vi "Config - Query.vi"(8 "error in (no error)":errorcluster, 11 "Config Records":T1[](array[typedef])) -> (0 "error out":errorcluster, 3 "Timing Data":u32[](array[numeric]))   [LabVIEW 2017]
doc: "Provide query timing data operation for configuration database process.\n[Covers: SD5]"
uses:
  Controls/Config Record.ctl
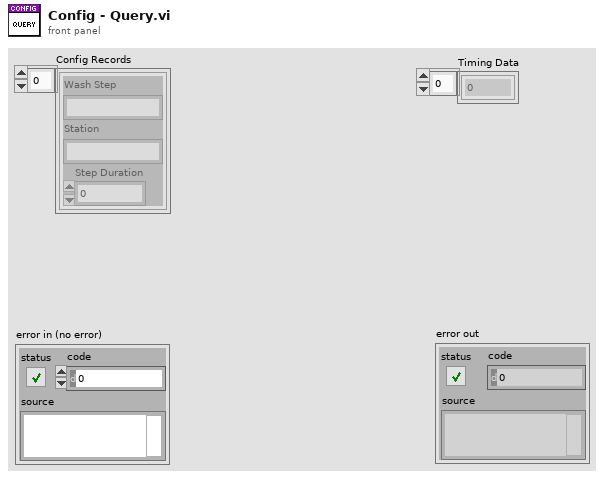
[diagram p1: front panel]
types:
  T1 = typedef "Config Record.ctl" = cluster{"Wash Step":string, "Station":string, "Step Duration":u32}
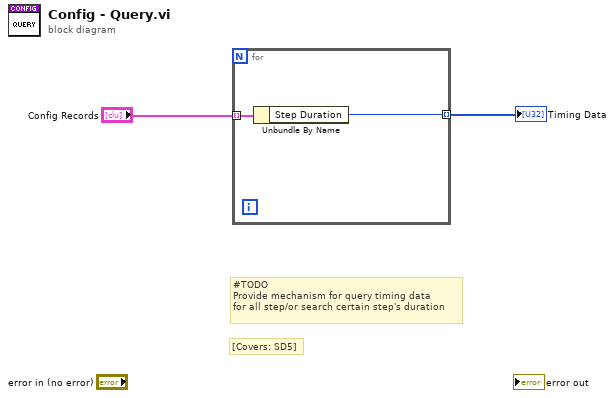
[diagram p0: block diagram]
diagram:
  # "[Covers: SD5]"
  # "#TODO\nProvide mechanism for query timing data\nfor all step/or search certain step's duration"
  n1 = for {
    tunnel: "Config Records" -> [w4] mode=indexing
    tunnel: [w3] -> w1 mode=indexing
    n2 = Unbundle By Name(w4) -> ("Step Duration"=w3:u32)
  }
  "Timing Data" <- w1
